vi "Read boolean in B.vi"(8 "error in (no error)":errorcluster, 11 "B in":refnum<class "B.lvclass">) -> (0 "error out":errorcluster, 2 "boolean in B":bool, 3 "B out":refnum<class "B.lvclass">)   [LabVIEW 2013, in "B.lvclass"]
uses:
  B.lvclass
  B.lvclass/B.ctl
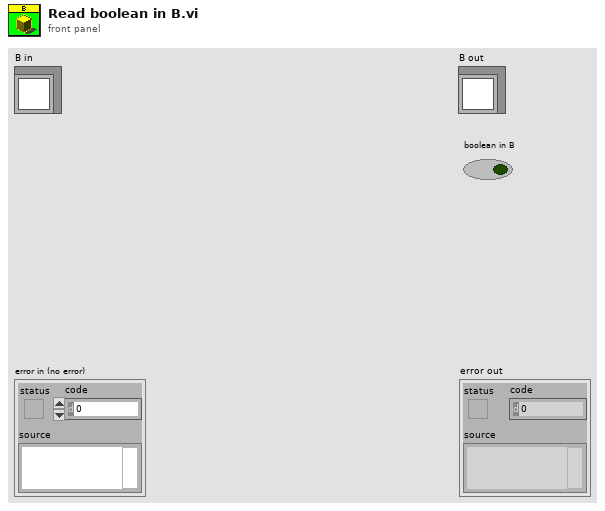
[diagram p1: front panel]
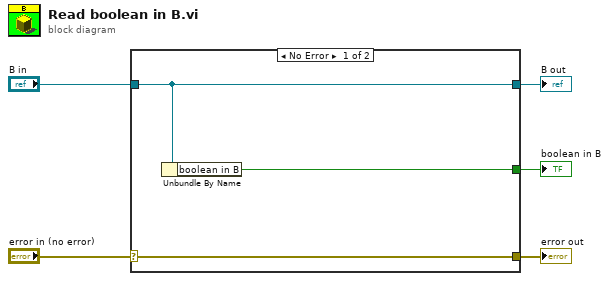
[diagram p0: block diagram]
diagram:
  n1 = case shown="No Error" "error in (no error)" {
    selector: "error in (no error)" -> [w8 w9]
    tunnel: [w8 w9] -> w4
    tunnel: [w7 w10] -> w2
    tunnel: "B in" -> [w7 w10]
    tunnel: [w6 _] -> w1
    frame No Error {
      n2 = Unbundle By Name(w7) -> ("boolean in B"=w6:bool)
    }
    frame Error {
    }
  }
  "error out" <- w4
  "B out" <- w2
  "boolean in B" <- w1
